vi "Parameters.vi"() -> ()   [LabVIEW 2019]
panel:
  in  "Information Section":T1={"Section"="People", "Control Properties"=[{"Label"="Name", "Data type"=enum."String"}, {"Label"="Age", "Data type"=enum."I32"}, {"Label"="Foreign?", "Data type"=enum."Boolean"}, {"Label"="Height", "Data type"=enum."Double"}]}
  in  "People Section":T1={"Section"="People", "Control Properties"=[{"Label"="Name", "Data type"=enum."String"}, {"Label"="Age", "Data type"=enum."I32"}, {"Label"="Foreign?", "Data type"=enum."Boolean"}, {"Label"="Height", "Data type"=enum."Double"}]}
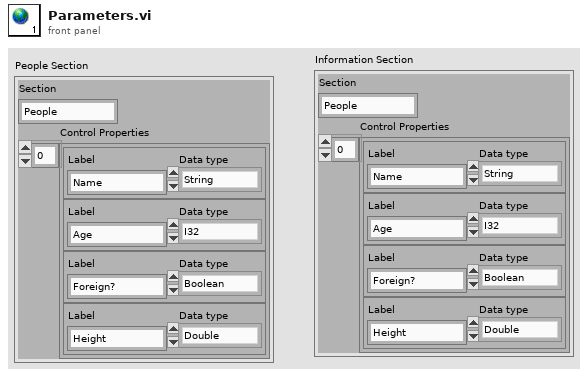
[diagram p1: front panel]
types:
  T1 = cluster{"Section":string, "Control Properties":cluster{"Label":string, "Data type":enum16{"Double", "I32", "Boolean", "String", "File Path"}}[]}
diagram:
